vi "Create.vi"(8 "error in (no error)":errorcluster, 10 "Input":string) -> (0 "error out":errorcluster, 3 "Proto":refnum<class "Group.lvclass">)   [LabVIEW 2020, in "Group.lvclass"]
uses:
  Group.lvclass
  Group.lvclass/Group.ctl
  Helpers/Helpers.lvlib
panel:
  out "Parsed Array 2":string[][](array[string])
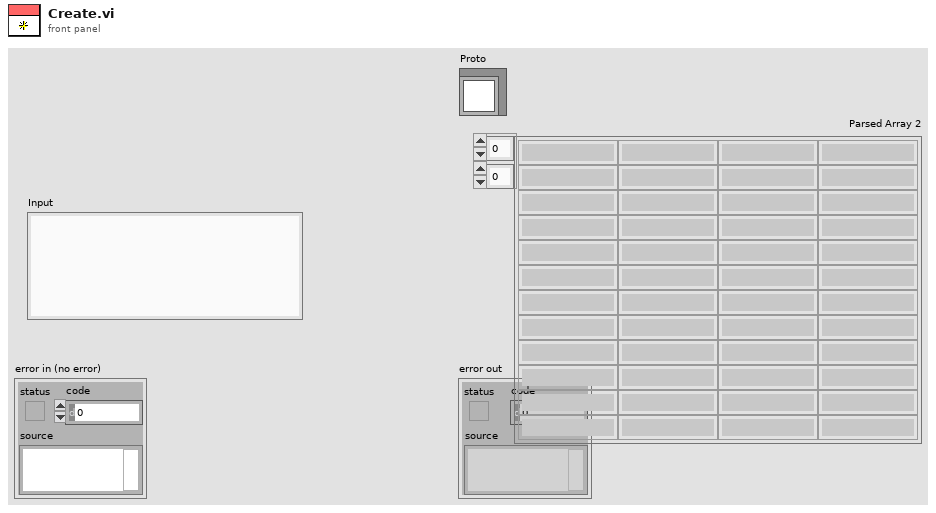
[diagram p1: front panel]
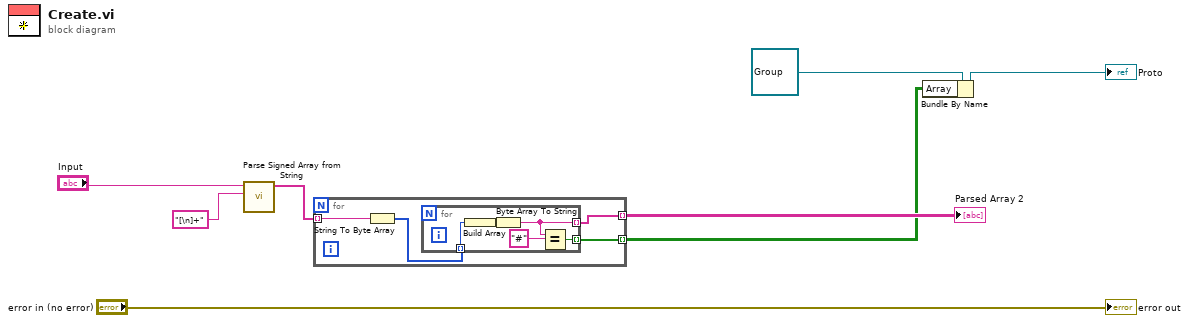
[diagram p0: block diagram]
diagram:
  n1 = call "Parse Signed Array from String.vi"("Delimiter regex"="[\n]+", "Input"="Input") -> ("Parsed Array"=w4:string[])  [unwired: 8 in, 1 out]
  n2 = for {
    tunnel: w4 -> [w12] mode=indexing
    tunnel: [w10] -> w3 mode=indexing
    tunnel: [w9] -> w1 mode=indexing
    n3 = String To Byte Array(string=w12) -> (unsigned byte array=w11:u8[])
    n4 = for {
      tunnel: w11 -> [w17] mode=indexing
      tunnel: [w15] -> w10 mode=indexing
      tunnel: [w13] -> w9 mode=indexing
      n5 = Build Array(w17) -> (w16:u8[])
      n6 = Byte Array To String(unsigned byte array=w16) -> (string=w15:string)
      n7 = Equal?(x=w15, y="#") -> (x = y?=w13:bool)
    }
  }
  "Parsed Array 2" <- w3
  n8 = Bundle By Name(cluster=refnum<class "Group.lvclass"> refnum ("Proto"), "Array"=w1) -> (→"Proto":refnum<class "Group.lvclass">)
  "error out" <- "error in (no error)"
